vi "get desired keys.vi"(8 "error in":errorcluster, 11 "Watchdog configuration in":refnum<class "Watchdog configuration.lvclass">) -> (0 "error out":errorcluster, 2 "desired keys":string[](array[string]), 3 "Watchdog configuration out":refnum<class "Watchdog configuration.lvclass">)   [LabVIEW 2013, in "Watchdog configuration.lvclass"]
uses:
  Watchdog configuration.lvclass
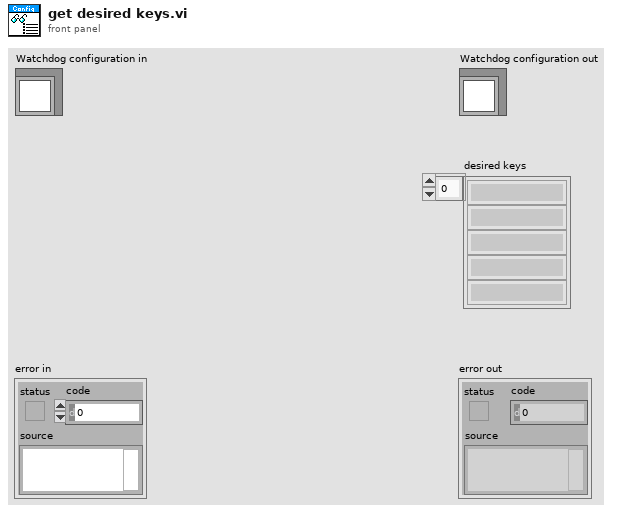
[diagram p1: front panel]
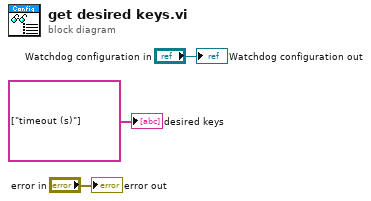
[diagram p0: block diagram]
diagram:
  "error out" <- "error in"
  "Watchdog configuration out" <- "Watchdog configuration in"
  "desired keys" <- string[] ["timeout (s)"] ("desired keys")
